vi "Clear.vi"(8 "error in (no error)":errorcluster, 11 "Character LCD in":refnum<class "OLED.lvclass">) -> (0 "error out":errorcluster, 2 "2D Picture":picture, 3 "Character LCD out":refnum<class "OLED.lvclass">)   [LabVIEW 2020, in "CTI-Peripheral.lvlib" / "OLED.lvclass"]
uses:
  OLED.lvclass
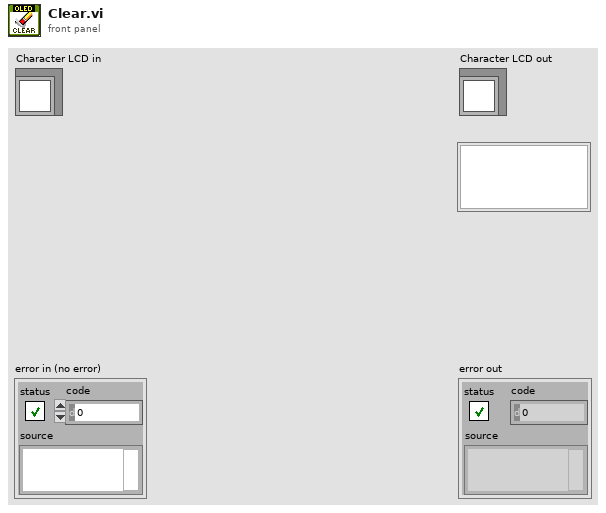
[diagram p1: front panel]
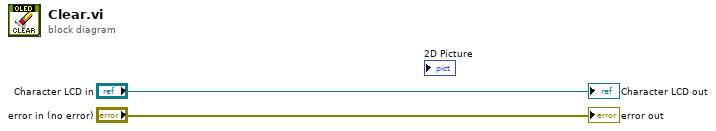
[diagram p0: block diagram]
diagram:
  "error out" <- "error in (no error)"
  "Character LCD out" <- "Character LCD in"
